vi "init.vi"(0 "Digital Input Test in":refnum<class "Test Pressure.lvclass">, 1 "ReadILCStrategy":refnum<class "IReadILCStrategy.lvclass">, 2 "ConfigureILCStrategy":refnum<class "IConfigureILCStrategy.lvclass">, 3 "Pressure Test":T1, 4 "Sample Delay":i32, 5 "error in (no error)":errorcluster, 6 "Test Scenario":T2, 7 "Log":refnum<class "ITestLog.lvclass">, 8 "Signal Name":string, 9 "Wait":i32, 10 "Samples To Read":i32) -> (14 "Digital Input Test out":refnum<class "Test Pressure.lvclass">, 19 "error out":errorcluster)   [LabVIEW 2015, in "Test Pressure.lvclass"]
uses:
  Test Pressure.lvclass
  Model/TestLog/ITestLog/ITestLog.lvclass
  Typedefs/TestScenarioTypes.ctl
  Model/ConfigureILCStrategy/IConfigureILCStrategy/IConfigureILCStrategy.lvclass
  Typedefs/Pressure Test.ctl
  Model/ReadILCStrategy/IReadILCStrategy/IReadILCStrategy.lvclass
  Test Pressure.lvclass/Test Pressure.ctl
  Typedefs/ILCBTTypedefs.lvlib
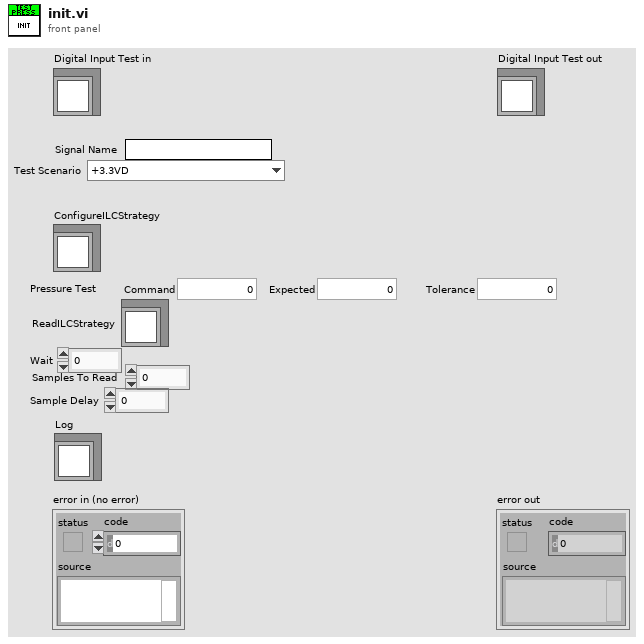
[diagram p1: front panel]
types:
  T1 = typedef "ILCBTTypedefs.lvlib/Pressure Test.ctl" = cluster{"Command":u16, "Expected":u16, "Tolerance":u16}
  T2 = typedef "ILCBTTypedefs.lvlib/TestScenarioTypes.ctl" = enum16{"+3.3VD", "+5.1V", "+24V", "RELVALV1", "RELVALV2", "Verify DAC_A = -1.00A", "Verify DAC_A = -0.75A", "Verify DAC_A = -0.50A", "Verify DAC_A = -0.25A", "Verify DAC_A = 0.00A", "Verify DAC_A = 0.25A", "Verify DAC_A = 0.50A", "Verify DAC_A = 0.75A", "Verify DAC_A = 1.00A", "Verify DAC_B = -1.00A", "Verify DAC_B = -0.75A", "Verify DAC_B = -0.50A", "Verify DAC_B = -0.25A", "Verify DAC_B = 0.00A", "Verify DAC_B = 0.25A", "Verify DAC_B = 0.50A", "Verify DAC_B = 0.75A", "Verify DAC_B = 1.00A", "Set DAC_A = -1.00A", "Set DAC_A = -0.75A", "Set DAC_A = -0.50A", "Set DAC_A = -0.25A", "Set DAC_A = 0.00A", "Set DAC_A = 0.25A", "Set DAC_A = 0.50A", "Set DAC_A = 0.75A", "Set DAC_A = 1.00A", "Set DAC_B = -1.00A", "Set DAC_B = -0.75A", "Set DAC_B = -0.50A", "Set DAC_B = -0.25A", "Set DAC_B = 0.00A", "Set DAC_B = 0.25A", "Set DAC_B = 0.50A", "Set DAC_B = 0.75A", "Set DAC_B = 1.00A", "Set MTR_PWR = On", "Set MTR_PWR = Off", "Set OUTPUT = On", "Set OUTPUT = Off", "Verify OUTPUT = On", "Verify OUTPUT = Off", "Verify POWER = Ok", "Verify POWER = Fail", "Verify AMP1 = Ok", "Verify AMP1 = Fail", "Verify AMP2 = Ok", "Verify AMP2 = Fail", "P1 0%", "P1 25%", "P1 50%", "P1 75%", "P1 100%", "P2 0%", "P2 25%", "P2 50%", "P2 75%", "P2 100%", "P3 0%", "P3 25%", "P3 50%", "P3 75%", "P3 100%", "P4 0%", "P4 25%", "P4 50%", "P4 75%", "P4 100%"}
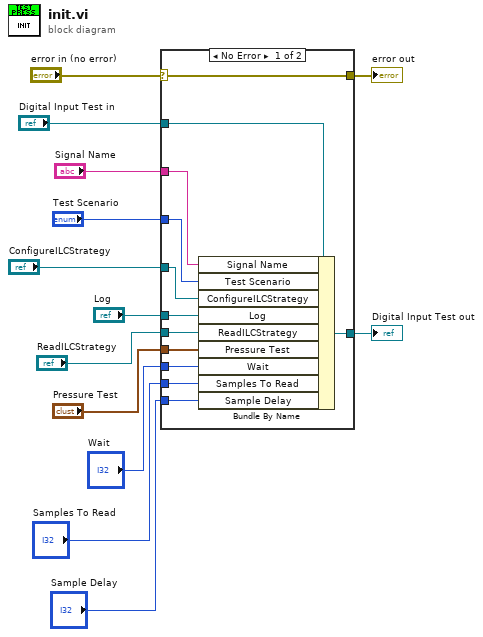
[diagram p0: block diagram]
diagram:
  n1 = case shown="No Error" "error in (no error)" {
    selector: "error in (no error)" -> [w25 w27]
    tunnel: [w25 w27] -> w12
    tunnel: [w21 w26] -> w10
    tunnel: "Digital Input Test in" -> [w24 w26]
    tunnel: "Signal Name" -> [w20 _]
    tunnel: "Test Scenario" -> [w19 _]
    tunnel: "ConfigureILCStrategy" -> [w22 _]
    tunnel: "Log" -> [w23 _]
    tunnel: "ReadILCStrategy" -> [w18 _]
    tunnel: "Wait" -> [w17 _]
    tunnel: "Pressure Test" -> [w16 _]
    tunnel: "Samples To Read" -> [w15 _]
    tunnel: "Sample Delay" -> [w14 _]
    frame No Error {
      n2 = Bundle By Name(cluster=w24, "Signal Name"=w20, "Test Scenario"=w19, "ConfigureILCStrategy"=w22, "Log"=w23, "ReadILCStrategy"=w18, "Pressure Test"=w16, "Wait"=w17, "Samples To Read"=w15, "Sample Delay"=w14) -> (w21:refnum<class "Test Pressure.lvclass">)
    }
    frame Error {
    }
  }
  "error out" <- w12
  "Digital Input Test out" <- w10
